vi "Get Description.vi"(11 "Condiment Decorator in":refnum<class "Condiment Decorator.lvclass">) -> (2 "Description":string, 3 "Condiment Decorator out":refnum<class "Condiment Decorator.lvclass">)   [LabVIEW 2011, in "Condiment Decorator.lvclass"]
uses:
  Condiment Decorator.lvclass
  Beverage/Beverage.lvclass
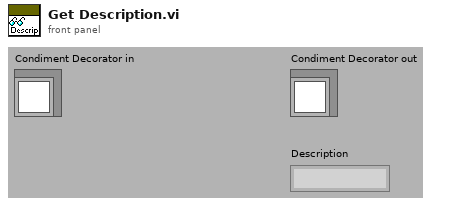
[diagram p1: front panel]
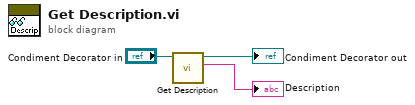
[diagram p0: block diagram]
diagram:
  n1 = call-parent "Get Description.vi"("Beverage in"="Condiment Decorator in") -> ("Description"=→"Description":string, "Beverage out"=→"Condiment Decorator out":refnum<class "Condiment Decorator.lvclass">)  [unwired: 9 in]
